vi "chaulin matador de porcos.vi"() -> ()   [LabVIEW 2020]
panel:
  in  "millisecond timer value":u32
  out "2 2":waveform(dbl)(graph)
  in  "stop":bool
  out "2":waveform(dbl)(graph)
  out "output waveform":waveform(dbl)
  out "1":waveform(dbl)(graph)
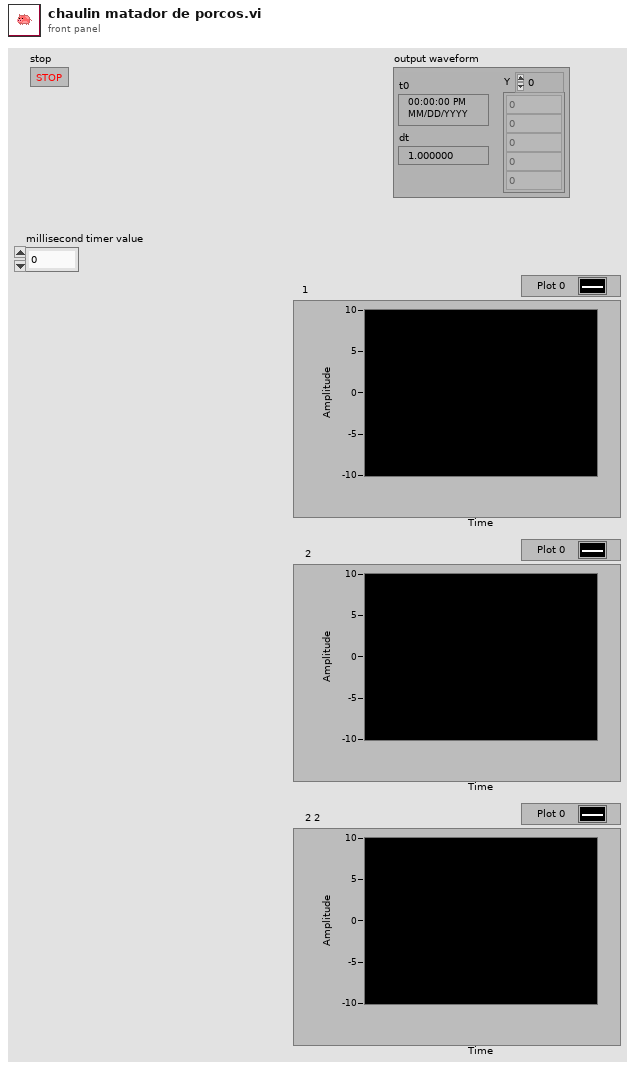
[diagram p1: front panel]
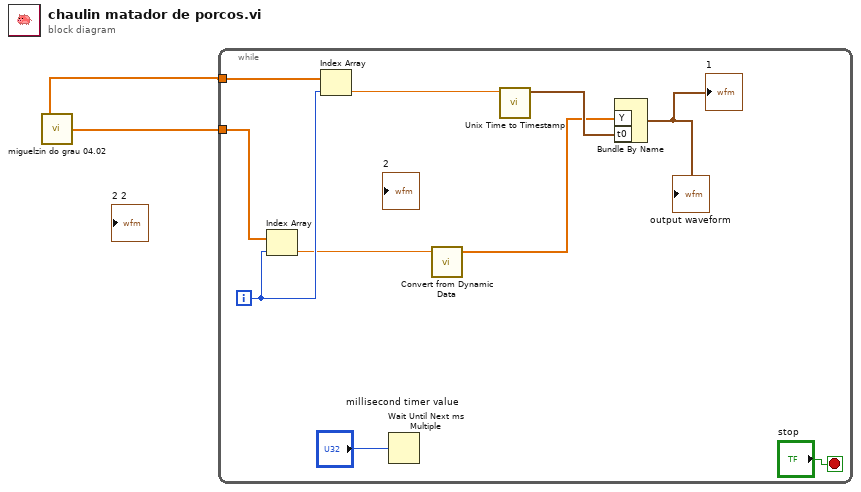
[diagram p0: block diagram]
diagram:
  n1 = call "miguelzin do grau 04.02.vi"() -> ("Timestamp"=w2:dbl[], "A"=w1:dbl[])  [unwired: 2 out]
  n2 = while {
    tunnel: w2 -> [w12]
    tunnel: w1 -> [w11]
    i -> [w10]
    stop <- "stop" stop-if-true
    n3 = Index Array(array=w12, index=w10) -> (element=w6:dbl)
    n4 = Index Array(array=w11, index=w10) -> (element=w9:dbl)
    n5 = Wait Until Next ms Multiple(millisecond multiple="millisecond timer value") -> ()  [unwired: 1 out]
    n6 = call "Convert from Dynamic Data"("Dynamic Data Type"=w6) -> ("Array"=w7:dbl[])  [unwired: 3 in]
    n7 = call <vilib>:"Unix Time to Timestamp.vi"("Unix Time (s)"=w9) -> ("Timestamp"=w8:timestamp)  [unwired: 9 in, 1 out]
    n8 = Bundle By Name("Y"=w7, "t0"=w8) -> (→"1" →"output waveform":waveform(dbl))  [unwired: 1 in]
  }
